vi "Results to Waveforms (array of doubles).vi"(1 "data type":dbl[][](array[numeric]), 7 "result references":T1[](array[typedef]), 11 "error in (no error)":errorcluster) -> (6 "signals out":dbl[][](array[numeric]), 8 "result references out":T1[](array[typedef]), 15 "error out":errorcluster)   [LabVIEW 2020, in "NI_DataFinder.lvlib"]
doc: "Extracts the signals from the results of a DataFinder search."
uses:
  <vilib>/DataFinder/NI_DataFinder.lvlib
  <vilib>/userdefined/DFSearchResult.ctl
  <vilib>/userdefined/NI_DataFinder Controls.lvlib
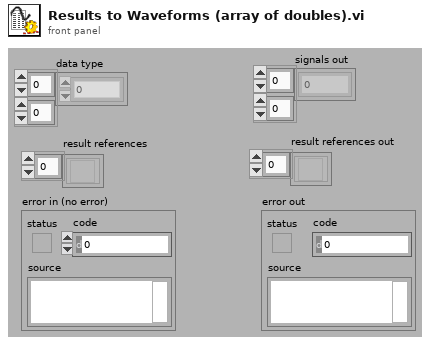
[diagram p1: front panel]
types:
  T1 = typedef "NI_DataFinder Controls.lvlib/DFSearchResult.ctl" = refnum<k20>
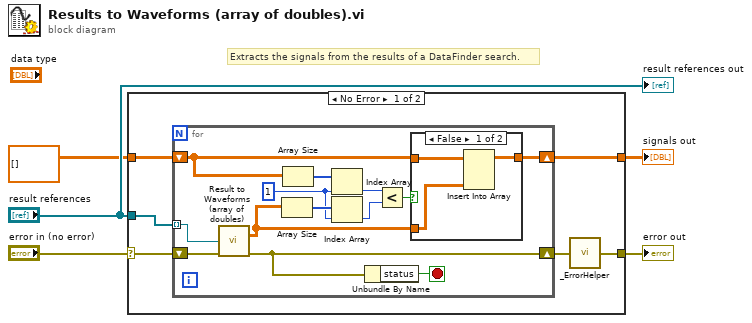
[diagram p0: block diagram]
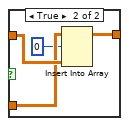
[diagram p2: hidden frame]
diagram:
  # "Extracts the signals from the results of a DataFinder search."
  n1 = case shown="No Error" "error in (no error)" {
    selector: "error in (no error)" -> [w7 w33]
    tunnel: "result references" -> [w11 _]
    tunnel: [w10 w32] -> w4
    tunnel: [w8 w33] -> w3
    tunnel: dbl[][] [] ("signals out") -> [w6 w32]
    frame No Error {
      n2 = for {
        shift-right: [w13] -> w10
        shift-left: w6 -> [w14]
        tunnel: w11 -> [w24] mode=indexing
        shift-right: [w22] -> w9
        shift-left: w7 -> [w23]
        stop <- w21 stop-if-true
        w18 = 1 ("index")
        n3 = call <vilib>:"Result to Waveforms (array of doubles).vi"("result reference"=w24, "error in"=w23) -> ("signals out"=w12:dbl[][], "error out"=w22:errorcluster)  [unwired: 1 in, 11 out]
        n4 = Array Size(array=w12) -> (size(s)=w19:i32[])
        n5 = Array Size(array=w14) -> (size(s)=w20:i32[])
        n6 = Index Array(array=w20, index=w18) -> (element=w16:i32)
        n7 = Index Array(array=w19, index=w18) -> (element=w17:i32)
        n8 = Unbundle By Name(w22) -> ("status"=w21:bool)
        n9 = Less?(x=w16, y=w17) -> (x < y?=w15:bool)
        n10 = case shown="False" w15 {
          tunnel: w14 -> [w26 w31]
          tunnel: w12 -> [w27 w30]
          tunnel: [w25 w28] -> w13
          frame False {
            n11 = Insert Into Array(array=w26, new element=w27) -> (w25:dbl[][])  [unwired: 2 in]
          }
          frame True {
            n12 = Insert Into Array(array=w30, index (row)=0, new element=w31) -> (w28:dbl[][])  [unwired: 1 in]
          }
        }
      }
      n13 = call <vilib>:"_ErrorHelper.vi"("error IO"=w9) -> ("error out"=w8:errorcluster)
    }
    frame Error {
    }
  }
  "error out" <- w3
  "signals out" <- w4
  "result references out" <- "result references"
